vi "DecodificaDO_new.vi"(0 "Array":T7[](array[typedef]), 7 "DO PLCs in":T5, 9 "statoDO Cdaq in":T9, 11 "DO interfaccia in":T6) -> (6 "Exit?":bool, 8 "DO PLCs out":T4, 10 "statoDO Cdaq out":T9, 15 "DO interfaccia out":T6)   [LabVIEW 2019]
uses:
  controls/statoDO_Cdaq.ctl
  cDAQ/SET SINGLE DO.ctl
  cDAQ/DO List.ctl
  TypeDef/DOinterfaccia.ctl
  ST1200_LIST_IO/StatoDO_PLC_1.ctl
  ST1200_LIST_IO/StatoDO_PLC_2.ctl
  ST1200_LIST_IO/StatoDO_PLC_3.ctl
  GlobalForzaUscite.vi
  Global_DO_Interfaccia.vi
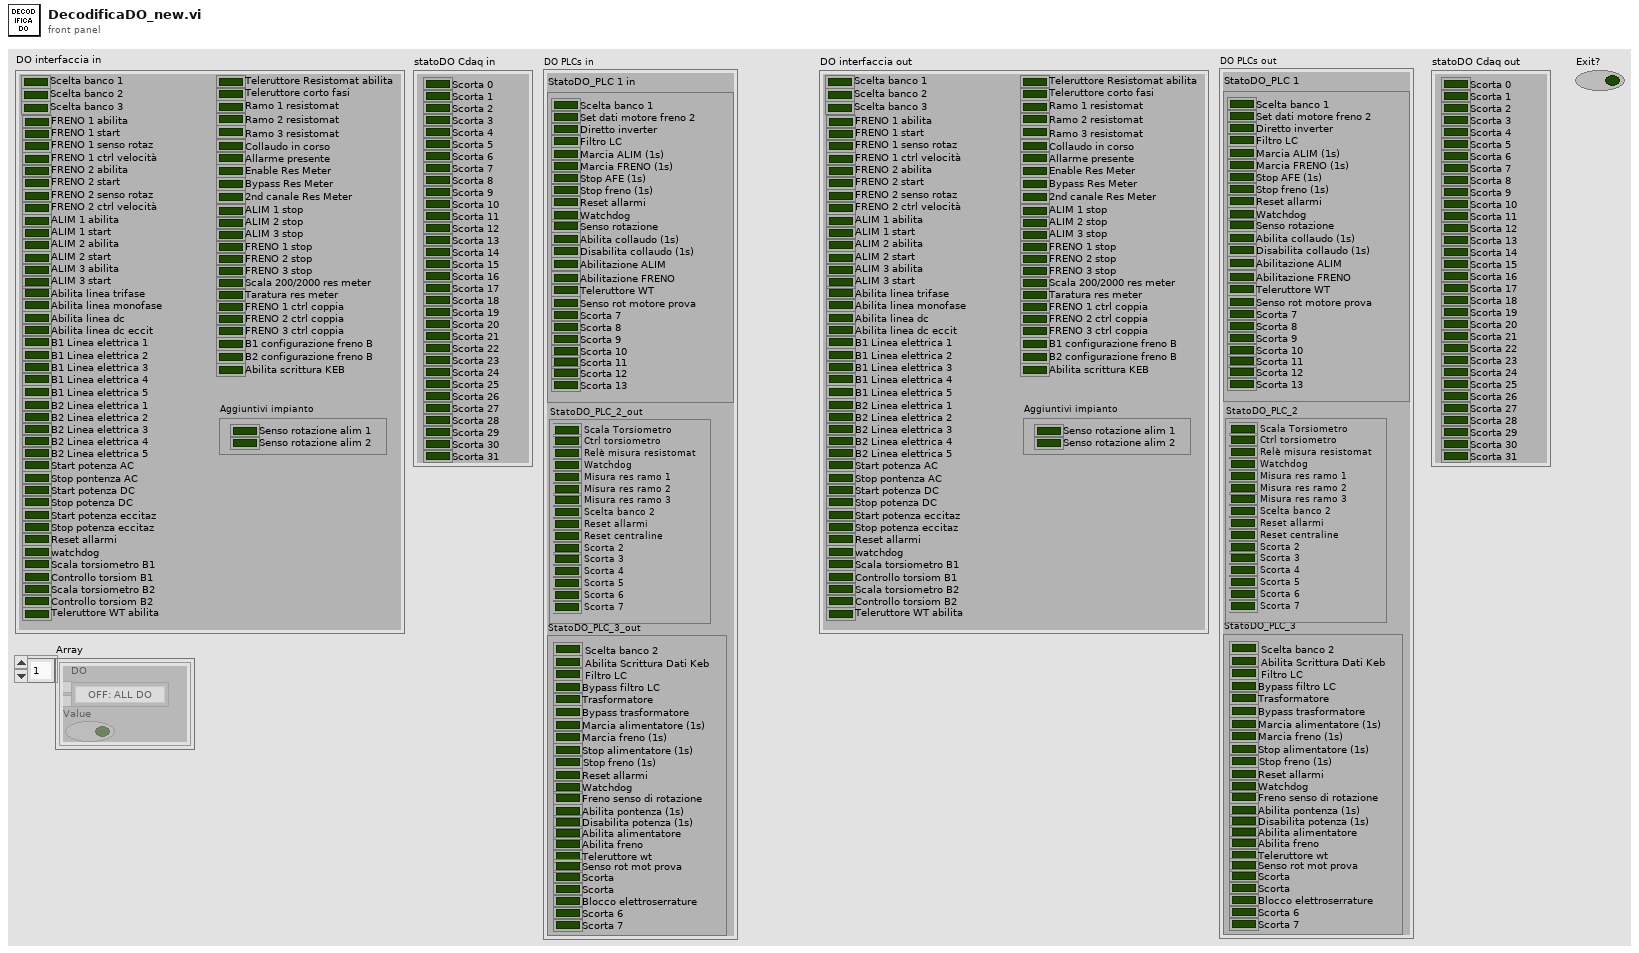
[diagram p1: front panel]
types:
  T1 = typedef "StatoDO_PLC_1.ctl" = cluster{"Scelta banco 1":bool, "Set dati motore freno 2":bool, "Diretto inverter":bool, "Filtro LC":bool, "Marcia ALIM (1s)":bool, "Marcia FRENO (1s)":bool, "Stop AFE (1s)":bool, "Stop freno (1s)":bool, "Reset allarmi":bool, "Watchdog":bool, "Senso rotazione":bool, "Abilita collaudo (1s)":bool, "Disabilita collaudo (1s)":bool, "Abilitazione ALIM":bool, "Abilitazione FRENO":bool, "Teleruttore WT":bool, "Senso rot motore prova":bool, "Scorta 7":bool, "Scorta 8":bool, "Scorta 9":bool, "Scorta 10":bool, "Scorta 11":bool, "Scorta 12":bool, "Scorta 13":bool}
  T2 = typedef "StatoDO_PLC_2.ctl" = cluster{"Scala Torsiometro":bool, "Ctrl torsiometro":bool, "Relè misura resistomat":bool, "Watchdog":bool, "Misura res ramo 1":bool, "Misura res ramo 2":bool, "Misura res ramo 3":bool, "Scelta banco 2":bool, "Reset allarmi":bool, "Reset centraline":bool, "Scorta 2":bool, "Scorta 3":bool, "Scorta 4":bool, "Scorta 5":bool, "Scorta 6":bool, "Scorta 7":bool}
  T3 = typedef "StatoDO_PLC_3.ctl" = cluster{"Scelta banco 2":bool, "Abilita Scrittura Dati Keb":bool, "Filtro LC":bool, "Bypass filtro LC":bool, "Trasformatore":bool, "Bypass trasformatore":bool, "Marcia alimentatore (1s)":bool, "Marcia freno (1s)":bool, "Stop alimentatore (1s)":bool, "Stop freno (1s)":bool, "Reset allarmi":bool, "Watchdog":bool, "Freno senso di rotazione":bool, "Abilita pontenza (1s)":bool, "Disabilita potenza (1s)":bool, "Abilita alimentatore":bool, "Abilita freno":bool, "Teleruttore wt":bool, "Senso rot mot prova":bool, "Scorta":bool, "Scorta":bool, "Blocco elettroserrature":bool, "Scorta 6":bool, "Scorta 7":bool}
  T4 = cluster{"StatoDO_PLC 1":T1, "StatoDO_PLC_2":T2, "StatoDO_PLC_3":T3}
  T5 = cluster{"StatoDO_PLC 1 in":T1, "StatoDO_PLC_2_out":T2, "StatoDO_PLC_3_out":T3}
  T6 = typedef "DOinterfaccia.ctl" = cluster{"Scelta banco 1":bool, "Scelta banco 2":bool, "Scelta banco 3":bool, "FRENO 1 abilita":bool, "FRENO 1 start":bool, "FRENO 1 senso rotaz":bool, "FRENO 1 ctrl velocità":bool, "FRENO 2 abilita":bool, "FRENO 2 start":bool, "FRENO 2 senso rotaz":bool, "FRENO 2 ctrl velocità":bool, "ALIM 1 abilita":bool, "ALIM 1 start":bool, "ALIM 2 abilita":bool, "ALIM 2 start":bool, "ALIM 3 abilita":bool, "ALIM 3 start":bool, "Abilita linea trifase":bool, "Abilita linea monofase":bool, "Abilita linea dc":bool, "Abilita linea dc eccit":bool, "B1 Linea elettrica 1":bool, "B1 Linea elettrica 2":bool, "B1 Linea elettrica 3":bool, "B1 Linea elettrica 4":bool, "B1 Linea elettrica 5":bool, "B2 Linea elettrica 1":bool, "B2 Linea elettrica 2":bool, "B2 Linea elettrica 3":bool, "B2 Linea elettrica 4":bool, "B2 Linea elettrica 5":bool, "Start potenza AC":bool, "Stop pontenza AC":bool, "Start potenza DC":bool, "Stop potenza DC":bool, "Start potenza eccitaz":bool, "Stop potenza eccitaz":bool, "Reset allarmi":bool, "watchdog":bool, "Scala torsiometro B1":bool, "Controllo torsiom B1":bool, "Scala torsiometro B2":bool, "Controllo torsiom B2":bool, "Teleruttore WT abilita":bool, "Teleruttore Resistomat abilita":bool, "Teleruttore corto fasi":bool, "Ramo 1 resistomat":bool, "Ramo 2 resistomat":bool, "Ramo 3 resistomat":bool, "Collaudo in corso":bool, "Allarme presente":bool, "Enable Res Meter":bool, "Bypass Res Meter":bool, "2nd canale Res Meter":bool, "Scala 200/2000 res meter":bool, "Taratura res meter":bool, "FRENO 1 ctrl coppia":bool, "FRENO 2 ctrl coppia":bool, "FRENO 3 ctrl coppia":bool, "Aggiuntivi impianto":cluster{"Senso rotazione alim 1":bool, "Senso rotazione alim 2":bool}, "ALIM 1 stop":bool, "ALIM 2 stop":bool, "ALIM 3 stop":bool, "FRENO 1 stop":bool, "FRENO 2 stop":bool, "FRENO 3 stop":bool, "B1 configurazione freno B":bool, "B2 configurazione freno B":bool, "Abilita scrittura KEB":bool}
  T7 = typedef "SET SINGLE DO.ctl" = cluster{"DO":T8, "Value":bool}
  T8 = typedef "DO List.ctl" = enum16{"OFF: ALL DO", "*ABILITA freno 1", "*ABILITA freno 2", "*ABILITA freno 3", "*START freno 1", "*START freno 2", "*START freno 3", "*STOP freno 1", "*STOP freno 3", "*STOP freno 2", "*Senso rot freno 1", "*Senso rot freno 2", "*Senso rot freno 3", "*Ctrl velocità freno 1", "*Ctrl velocità freno 2", "*Ctrl velocità freno 3", "*Ctrl coppia freno 1", "*Ctrl coppia freno 2", "*Ctrl coppia freno 3", "*ABILITA alimentatore 1", "*ABILITA alimentatore 2", "*ABILITA alimentatore 3", "*ABILITA alimentatore 4", "*START alimentatore 1", "*START alimentatore 2", "*START alimentatore 3", "*START alimentatore 4", "*STOP alimentatore 1", "*STOP alimentatore 2", "*STOP alimentatore 3", "*STOP alimentatore 4", "SENSO ROT alimentatore 1", "SENSO ROT alimentatore 2", "Abilita LEM 1000A", "Abilita LEM 300A", "Abilita sensori EXT WT", "B1 Seleziona linea 1", "B1 Seleziona linea 2", "B1 Seleziona linea 3", "B1 Seleziona linea 4", "B1 Seleziona linea 5", "B2 Seleziona linea 1", "B2 Seleziona linea 2", "B2 Seleziona linea 3", "B2 Seleziona linea 4", "B2 Seleziona linea 5", "*Reset allarmi", "*Start potenza AC", "*Stop potenza AC", "*Start potenza DC", "*Stop potenza DC", "*Start potenza DC eccit", "*Stop pontenza DC eccit", "Bypass res meter", "2nd canale res meter", "Enable res meter", "*Abilit teler ramo WT", "*Abil teler ramo princ Resit", "*Abil teler ramo 1 Resist", "*Abil teler ramo 2 Resist", "*Abil teler ramo 3 Resist", "*Abil cortocirc avvolgim", "*Controllo torsiometro B1", "*Controllo Torsiom B2", "*Scala torsiometro B1", "*Scala torsiometro B2", "*Collaudo in corso", "*Allarme presente", "Abilitazione elettroserratura", "Exit", "*Abilita collaudo", "*Abilita potenza trifase", "*Abilita potenza monofase", "*Abilita potenza DC", "*Abilita potenza DC eccit", "*Disabilita teleruttori potenza", "Set teleruttori prova a freddo", "Prova a freddo monofase", "Watchdog", "Forza DO PLC 3", "Forza DO PLC 2", "Forza DO PLC 1", "Forza DO cDAQ", "Scala 2000(T) 200(F) res meter", "Seleziona banco 1", "Seleziona banco 2", "Comando azionam in blocco", "Comando azionam reset", "Sensibilità freno 16 32 nm", "Reset Allarmi", "Carico res - Ramo 1", "Carico res - Ramo 2", "Carico res - Ramo 3", "Carico res - Ramo 4", "Carico res - Ramo 5", "Carico res - Ramo 6", "Carico res - Ramo 7", "Carico res - Ramo 8", "Carico res - Ramo 9", "Carico res - Ramo 10", "Carico res - Ramo 11", "Carico res - Start ventilatore", "Carico res - Stop ventilatore", "Abilita potenza solo freno", "Abilita AFE + freno trasc", "Abilita potenza carico resistivo", "Chiudi potenza AFE", "Apri potenza AFE", "Start AFE", "Config Banco2 TDE", "Misura diretto WT", "Ripristina centralina protezioni", "Abilita Scrittura Dati Keb"}
  T9 = typedef "statoDO_Cdaq.ctl" = cluster{"Scorta 0":bool, "Scorta 1":bool, "Scorta 2":bool, "Scorta 3":bool, "Scorta 4":bool, "Scorta 5":bool, "Scorta 6":bool, "Scorta 7":bool, "Scorta 8":bool, "Scorta 9":bool, "Scorta 10":bool, "Scorta 11":bool, "Scorta 12":bool, "Scorta 13":bool, "Scorta 14":bool, "Scorta 15":bool, "Scorta 16":bool, "Scorta 17":bool, "Scorta 18":bool, "Scorta 19":bool, "Scorta 20":bool, "Scorta 21":bool, "Scorta 22":bool, "Scorta 23":bool, "Scorta 24":bool, "Scorta 25":bool, "Scorta 26":bool, "Scorta 27":bool, "Scorta 28":bool, "Scorta 29":bool, "Scorta 30":bool, "Scorta 31":bool}
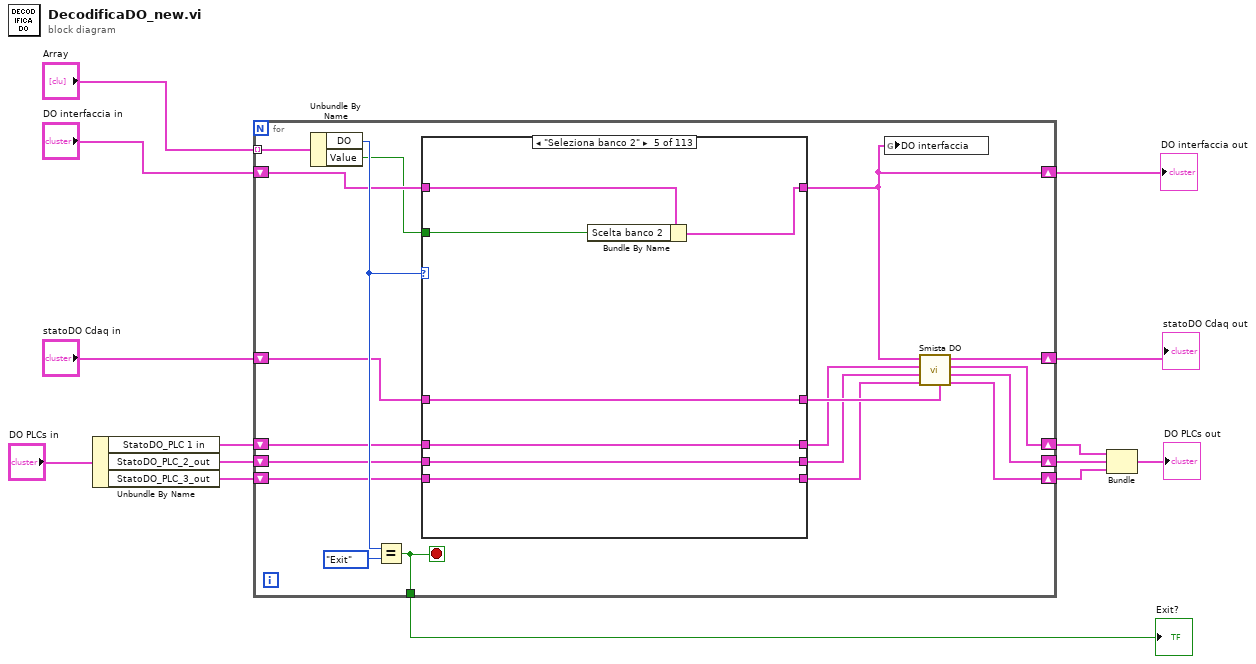
[diagram p0: block diagram]
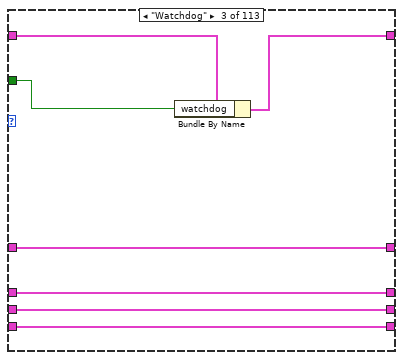
[diagram p4: hidden frame]
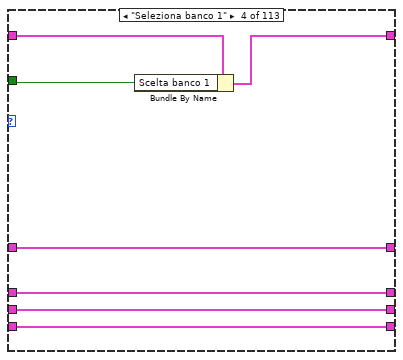
[diagram p5: hidden frame]
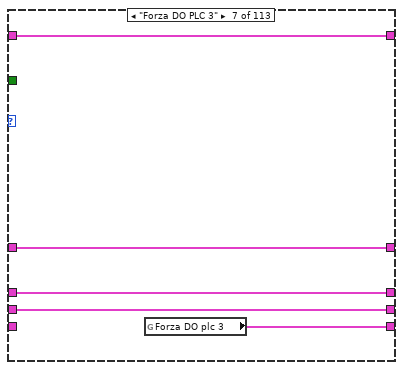
[diagram p7: hidden frame]
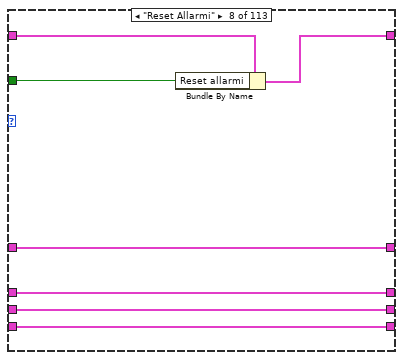
[diagram p8: hidden frame]
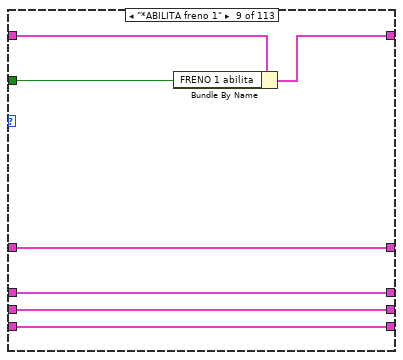
[diagram p9: hidden frame]
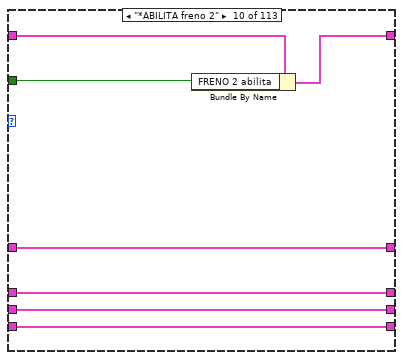
[diagram p10: hidden frame]
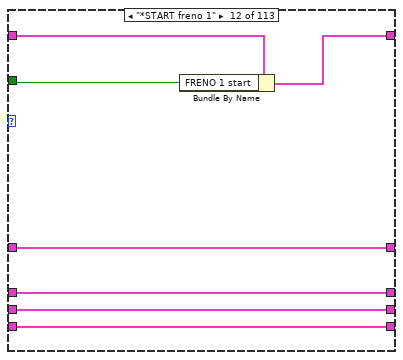
[diagram p12: hidden frame]
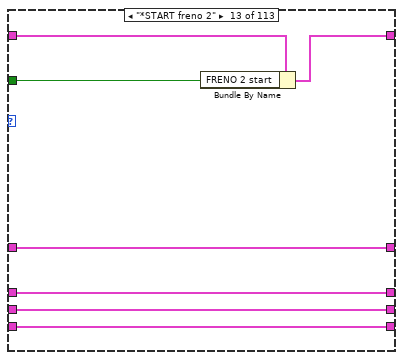
[diagram p13: hidden frame]
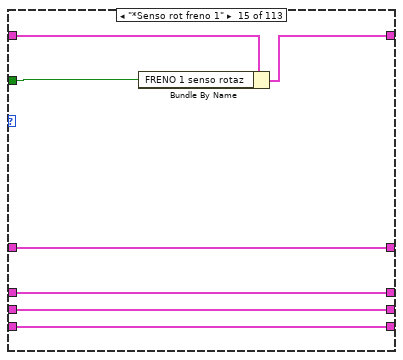
[diagram p15: hidden frame]
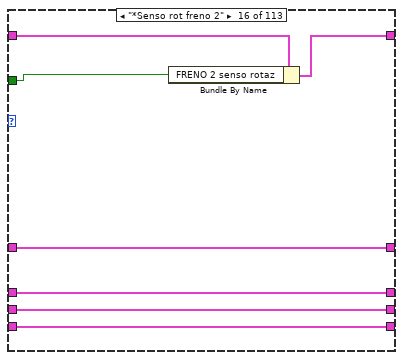
[diagram p16: hidden frame]
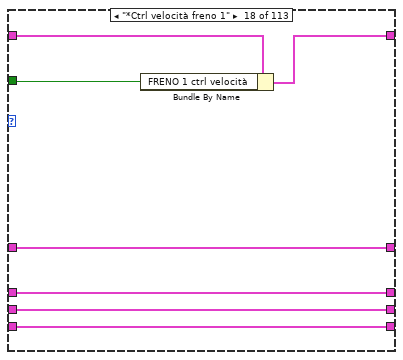
[diagram p18: hidden frame]
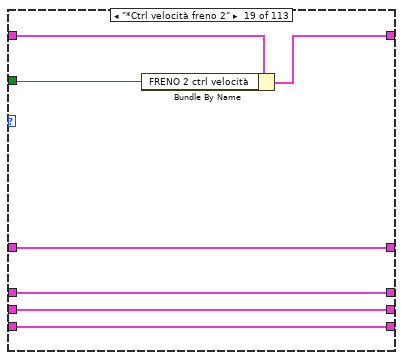
[diagram p19: hidden frame]
diagram:
  n1 = Unbundle By Name("DO PLCs in") -> ("StatoDO_PLC 1 in"=w7:T1, "StatoDO_PLC_2_out"=w6:T2, "StatoDO_PLC_3_out"=w5:T3)
  n2 = for {
    tunnel: "Array" -> [w33] mode=indexing
    shift-right: [w30] -> w11
    shift-left: "statoDO Cdaq in" -> [w24]
    tunnel: [w32] -> w14
    shift-right: [w22] -> w4
    shift-left: w7 -> [w25]
    shift-right: [w23] -> w9
    shift-left: "DO interfaccia in" -> [w27]
    shift-right: [w20] -> w3
    shift-left: w6 -> [w17]
    shift-right: [w19] -> w2
    shift-left: w5 -> [w18]
    stop <- w32 stop-if-true
    n3 = Unbundle By Name(w33) -> ("DO"=w29:T8, "Value"=w26:bool)
    n4 = Equal?(x=w29, y=DO_List."Exit" ("DO")) -> (x = y?=w32:bool)
    n5 = case shown="\"Seleziona banco 2\"" w29 {
      tunnel: [w37 w42 w49 w56 w63 w68 w71 w80 w87 w94 w99 w106 w113 w118 w125 w132 w137 w144 w151 w156 w163 w170 w177 w182 w189 w196 w203 w208 w216 w224 w232 w240 w248 w255 w262 w269 w276 w283 w288 w293 w300 w307 w314 w321 w328 w335 w342 w349 w356 w363 w370 w377 w384 w389 w394 w402 w410 w418 w426 w433 w441 w446 w453 w460 w467 w474 w481 w488 w493 w498 w503 w508 w509 w518 w523 w528 w533 w538 w543 w548 w553 w558 w563 w568 w575 w580 w585 w590 w595 w600 w605 w610 w615 w622 w627 w632 w639 w646 w653 w660 w667 w674 w681 w688 w693 w700 w707 w715 w723 w731 w739 w747 w754] -> w28
      tunnel: [w36 w41 w48 w55 w62 w67 w69 w79 w86 w93 w98 w105 w112 w117 w124 w131 w136 w143 w150 w155 w162 w169 w176 w181 w188 w195 w202 w207 w215 w223 w231 w239 w247 w254 w261 w268 w275 w282 w287 w292 w299 w306 w313 w320 w327 w334 w341 w348 w355 w362 w369 w376 w383 w388 w393 w401 w409 w417 w425 w432 w440 w445 w452 w459 w466 w473 w480 w487 w492 w497 w502 w504 w513 w517 w522 w527 w532 w537 w542 w547 w552 w557 w562 w567 w574 w579 w584 w589 w594 w599 w604 w609 w614 w621 w626 w631 w638 w645 w652 w659 w666 w673 w680 w687 w692 w699 w706 w714 w722 w730 w738 w746 w753] -> w21
      tunnel: [_ w40 w46 w53 w58 w64 w73 w77 w83 w91 w97 w102 w110 w116 w122 w129 w135 w141 w148 w154 w160 w167 w174 w180 w186 w193 w200 w206 w213 w220 w229 w237 w245 w252 w259 w264 w273 w278 w284 w289 w297 w304 w311 w318 w325 w332 w339 w345 w353 w360 w366 w374 w381 w385 w392 w399 w405 w413 w421 w430 w438 w444 w450 w457 w464 w470 w478 w485 w489 w494 w501 w507 w512 w514 w519 w524 w529 w534 w539 w544 w549 w554 w559 w564 w570 w576 w581 w586 w591 w596 w601 w606 w611 w616 w623 w628 w634 w641 w647 w655 w662 w668 w675 w682 w691 w695 w702 w710 w718 w726 w734 w742 w748] -> w23
      tunnel: w27 -> [_ w40 w47 w54 w59 w64 w73 w78 w85 w92 w97 w103 w111 w116 w123 w130 w135 w142 w149 w154 w161 w168 w175 w180 w187 w194 w201 w206 w214 w221 w230 w238 w246 w253 w260 w265 w274 w279 w284 w289 w298 w305 w312 w319 w326 w333 w340 w346 w354 w361 w367 w375 w382 w385 w392 w400 w406 w414 w422 w431 w439 w444 w451 w458 w465 w471 w479 w486 w489 w494 w501 w507 w512 w514 w519 w524 w529 w534 w539 w544 w549 w554 w559 w564 w571 w576 w581 w586 w591 w596 w601 w606 w611 w617 w623 w628 w635 w642 w649 w656 w663 w670 w676 w683 w691 w696 w703 w711 w719 w727 w735 w743 w750]
      tunnel: w26 -> [_ _ w45 w52 w57 _ _ w74 w84 w90 _ w104 w109 _ w121 w128 _ w140 w147 _ w159 w166 w173 _ w185 w192 w199 _ w212 w222 w228 w236 w244 w249 w258 w263 w272 w277 _ _ w296 w303 w310 w317 w324 w331 w338 w347 w352 w359 w368 w373 w380 _ _ w398 w404 w412 w420 _ _ _ w449 w456 w463 w472 w477 w484 _ _ _ _ _ _ _ _ _ _ _ _ _ _ _ _ _ _ _ _ _ _ _ _ _ w618 _ _ w633 w640 w648 w654 w661 w669 w677 w684 _ w694 w701 w709 w716 w724 w732 w740 w749]
      tunnel: w25 -> [w36 w41 w48 w55 w62 w67 w69 w79 w86 w93 w98 w105 w112 w117 w124 w131 w136 w143 w150 w155 w162 w169 w176 w181 w188 w195 w202 w207 w215 w223 w231 w239 w247 w254 w261 w268 w275 w282 w287 w292 w299 w306 w313 w320 w327 w334 w341 w348 w355 w362 w369 w376 w383 w388 w393 w401 w409 w417 w425 w432 w440 w445 w452 w459 w466 w473 w480 w487 w492 w497 w502 _ w513 w517 w522 w527 w532 w537 w542 w547 w552 w557 w562 w567 w574 w579 w584 w589 w594 w599 w604 w609 w614 w621 w626 w631 w638 w645 w652 w659 w666 w673 w680 w687 w692 w699 w706 w714 w722 w730 w738 w746 w753]
      tunnel: w24 -> [w37 w42 w49 w56 w63 w68 w71 w80 w87 w94 w99 w106 w113 w118 w125 w132 w137 w144 w151 w156 w163 w170 w177 w182 w189 w196 w203 w208 w216 w224 w232 w240 w248 w255 w262 w269 w276 w283 w288 w293 w300 w307 w314 w321 w328 w335 w342 w349 w356 w363 w370 w377 w384 w389 w394 w402 w410 w418 w426 w433 w441 w446 w453 w460 w467 w474 w481 w488 w493 w498 w503 w508 _ w518 w523 w528 w533 w538 w543 w548 w553 w558 w563 w568 w575 w580 w585 w590 w595 w600 w605 w610 w615 w622 w627 w632 w639 w646 w653 w660 w667 w674 w681 w688 w693 w700 w707 w715 w723 w731 w739 w747 w754]
      tunnel: w18 -> [w34 w38 w43 w50 w60 w65 _ w75 w81 w88 w95 w100 w107 w114 w119 w126 w133 w138 w145 w152 w157 w164 w171 w178 w183 w190 w197 w204 w209 w217 w225 w233 w241 w250 w256 w266 w270 w280 w285 w290 w294 w301 w308 w315 w322 w329 w336 w343 w350 w357 w364 w371 w378 w386 w390 w396 w407 w415 w423 w428 w434 w442 w447 w454 w461 w468 w475 w482 w490 w495 w500 w505 w510 w515 w520 w525 w530 w535 w540 w545 w550 w555 w560 w565 w572 w577 w582 w587 w592 w597 w602 w607 w612 w619 w624 w629 w636 w643 w650 w657 w664 w671 w678 w685 w689 w697 w704 w712 w720 w728 w736 w744 w751]
      tunnel: w17 -> [w35 w39 w44 w51 w61 w66 w72 w76 w82 w89 w96 w101 w108 w115 w120 w127 w134 w139 w146 w153 w158 w165 w172 w179 w184 w191 w198 w205 w210 w218 w226 w234 w242 w251 w257 w267 w271 w281 w286 w291 w295 w302 w309 w316 w323 w330 w337 w344 w351 w358 w365 w372 w379 w387 w391 w397 w408 w416 w424 w429 w435 w443 w448 w455 w462 w469 w476 w483 w491 w496 _ w506 w511 w516 w521 w526 w531 w536 w541 w546 w551 w556 w561 w566 w573 w578 w583 w588 w593 w598 w603 w608 w613 w620 w625 w630 w637 w644 w651 w658 w665 w672 w679 w686 w690 w698 w705 w713 w721 w729 w737 w745 w752]
      tunnel: [w35 w39 w44 w51 w61 w66 w72 w76 w82 w89 w96 w101 w108 w115 w120 w127 w134 w139 w146 w153 w158 w165 w172 w179 w184 w191 w198 w205 w210 w218 w226 w234 w242 w251 w257 w267 w271 w281 w286 w291 w295 w302 w309 w316 w323 w330 w337 w344 w351 w358 w365 w372 w379 w387 w391 w397 w408 w416 w424 w429 w435 w443 w448 w455 w462 w469 w476 w483 w491 w496 w499 w506 w511 w516 w521 w526 w531 w536 w541 w546 w551 w556 w561 w566 w573 w578 w583 w588 w593 w598 w603 w608 w613 w620 w625 w630 w637 w644 w651 w658 w665 w672 w679 w686 w690 w698 w705 w713 w721 w729 w737 w745 w752] -> w16
      tunnel: [w34 w38 w43 w50 w60 w65 w70 w75 w81 w88 w95 w100 w107 w114 w119 w126 w133 w138 w145 w152 w157 w164 w171 w178 w183 w190 w197 w204 w209 w217 w225 w233 w241 w250 w256 w266 w270 w280 w285 w290 w294 w301 w308 w315 w322 w329 w336 w343 w350 w357 w364 w371 w378 w386 w390 w396 w407 w415 w423 w428 w434 w442 w447 w454 w461 w468 w475 w482 w490 w495 w500 w505 w510 w515 w520 w525 w530 w535 w540 w545 w550 w555 w560 w565 w572 w577 w582 w587 w592 w597 w602 w607 w612 w619 w624 w629 w636 w643 w650 w657 w664 w671 w678 w685 w689 w697 w704 w712 w720 w728 w736 w744 w751] -> w15
      frame "OFF: ALL DO", Default {
      }
      frame "Exit" {
      }
      frame "Watchdog" {
        n6 = Bundle By Name(cluster=w47, "watchdog"=w45) -> (w46:T6)
      }
      frame "Seleziona banco 1" {
        n7 = Bundle By Name(cluster=w54, "Scelta banco 1"=w52) -> (w53:T6)
      }
      frame "Seleziona banco 2" {
        n8 = Bundle By Name(cluster=w59, "Scelta banco 2"=w57) -> (w58:T6)
      }
      frame "Comando azionam in blocco" {
      }
      frame "Forza DO PLC 3" {
        n9 = global read "GlobalForzaUscite.vi" "Forza DO plc 3"() -> (w70:T3)
      }
      frame "Reset Allarmi" {
        n10 = Bundle By Name(cluster=w78, "Reset allarmi"=w74) -> (w77:T6)
      }
      frame "*ABILITA freno 1" {
        n11 = Bundle By Name(cluster=w85, "FRENO 1 abilita"=w84) -> (w83:T6)
      }
      frame "*ABILITA freno 2" {
        n12 = Bundle By Name(cluster=w92, "FRENO 2 abilita"=w90) -> (w91:T6)
      }
      frame "*ABILITA freno 3" {
      }
      frame "*START freno 1" {
        n13 = Bundle By Name(cluster=w103, "FRENO 1 start"=w104) -> (w102:T6)
      }
      frame "*START freno 2" {
        n14 = Bundle By Name(cluster=w111, "FRENO 2 start"=w109) -> (w110:T6)
      }
      frame "*START freno 3" {
      }
      frame "*Senso rot freno 1" {
        n15 = Bundle By Name(cluster=w123, "FRENO 1 senso rotaz"=w121) -> (w122:T6)
      }
      frame "*Senso rot freno 2" {
        n16 = Bundle By Name(cluster=w130, "FRENO 2 senso rotaz"=w128) -> (w129:T6)
      }
      frame "*Senso rot freno 3" {
      }
      frame "*Ctrl velocità freno 1" {
        n17 = Bundle By Name(cluster=w142, "FRENO 1 ctrl velocità"=w140) -> (w141:T6)
      }
      frame "*Ctrl velocità freno 2" {
        n18 = Bundle By Name(cluster=w149, "FRENO 2 ctrl velocità"=w147) -> (w148:T6)
      }
      frame "*Ctrl velocità freno 3" {
      }
      frame "*ABILITA alimentatore 1" {
        n19 = Bundle By Name(cluster=w161, "ALIM 1 abilita"=w159) -> (w160:T6)
      }
      frame "*ABILITA alimentatore 2" {
        n20 = Bundle By Name(cluster=w168, "ALIM 2 abilita"=w166) -> (w167:T6)
      }
      frame "*ABILITA alimentatore 3" {
        n21 = Bundle By Name(cluster=w175, "ALIM 3 abilita"=w173) -> (w174:T6)
      }
      frame "*ABILITA alimentatore 4" {
      }
      frame "*START alimentatore 1" {
        n22 = Bundle By Name(cluster=w187, "ALIM 1 start"=w185) -> (w186:T6)
      }
      frame "*START alimentatore 2" {
        n23 = Bundle By Name(cluster=w194, "ALIM 2 start"=w192) -> (w193:T6)
      }
      frame "*START alimentatore 3" {
        n24 = Bundle By Name(cluster=w201, "ALIM 3 start"=w199) -> (w200:T6)
      }
      frame "*START alimentatore 4" {
      }
      frame "B1 Seleziona linea 1" {
        w211 = FALSE ("Linea elettrica 5")
        n25 = Bundle By Name(cluster=w214, "B1 Linea elettrica 1"=w212, "B1 Linea elettrica 2"=w211, "B1 Linea elettrica 3"=w211, "B1 Linea elettrica 4"=w211, "B1 Linea elettrica 5"=w211) -> (w213:T6)
      }
      frame "B1 Seleziona linea 2" {
        w219 = FALSE ("Linea elettrica 1")
        n26 = Bundle By Name(cluster=w221, "B1 Linea elettrica 1"=w219, "B1 Linea elettrica 2"=w222, "B1 Linea elettrica 3"=w219, "B1 Linea elettrica 4"=w219, "B1 Linea elettrica 5"=w219) -> (w220:T6)
      }
      frame "B1 Seleziona linea 3" {
        w227 = FALSE ("Linea elettrica 1")
        n27 = Bundle By Name(cluster=w230, "B1 Linea elettrica 1"=w227, "B1 Linea elettrica 2"=w227, "B1 Linea elettrica 3"=w228, "B1 Linea elettrica 4"=w227, "B1 Linea elettrica 5"=w227) -> (w229:T6)
      }
      frame "B1 Seleziona linea 4" {
        w235 = FALSE ("Linea elettrica 5")
        n28 = Bundle By Name(cluster=w238, "B1 Linea elettrica 1"=w235, "B1 Linea elettrica 2"=w235, "B1 Linea elettrica 3"=w235, "B1 Linea elettrica 4"=w236, "B1 Linea elettrica 5"=w235) -> (w237:T6)
      }
      frame "B1 Seleziona linea 5" {
        w243 = FALSE ("Linea elettrica 1")
        n29 = Bundle By Name(cluster=w246, "B1 Linea elettrica 1"=w243, "B1 Linea elettrica 2"=w243, "B1 Linea elettrica 3"=w243, "B1 Linea elettrica 4"=w243, "B1 Linea elettrica 5"=w244) -> (w245:T6)
      }
      frame "*Reset allarmi" {
        n30 = Bundle By Name(cluster=w253, "Reset allarmi"=w249) -> (w252:T6)
      }
      frame "*Start potenza AC" {
        n31 = Bundle By Name(cluster=w260, "Start potenza AC"=w258) -> (w259:T6)
      }
      frame "*Stop potenza AC" {
        n32 = Bundle By Name(cluster=w265, "Stop pontenza AC"=w263) -> (w264:T6)
      }
      frame "*Start potenza DC" {
        n33 = Bundle By Name(cluster=w274, "Start potenza DC"=w272) -> (w273:T6)
      }
      frame "*Stop potenza DC" {
        n34 = Bundle By Name(cluster=w279, "Stop potenza DC"=w277) -> (w278:T6)
      }
      frame "*Start potenza DC eccit" {
      }
      frame "*Stop pontenza DC eccit" {
      }
      frame "Bypass res meter" {
        n35 = Bundle By Name(cluster=w298, "Bypass Res Meter"=w296) -> (w297:T6)
      }
      frame "*Abilit teler ramo WT" {
        n36 = Bundle By Name(cluster=w305, "Teleruttore WT abilita"=w303) -> (w304:T6)
      }
      frame "*Abil teler ramo princ Resit" {
        n37 = Bundle By Name(cluster=w312, "Teleruttore Resistomat abilita"=w310) -> (w311:T6)
      }
      frame "*Abil teler ramo 1 Resist" {
        n38 = Bundle By Name(cluster=w319, "Ramo 1 resistomat"=w317) -> (w318:T6)
      }
      frame "*Abil teler ramo 2 Resist" {
        n39 = Bundle By Name(cluster=w326, "Ramo 2 resistomat"=w324) -> (w325:T6)
      }
      frame "*Abil teler ramo 3 Resist" {
        n40 = Bundle By Name(cluster=w333, "Ramo 3 resistomat"=w331) -> (w332:T6)
      }
      frame "*Abil cortocirc avvolgim" {
        n41 = Bundle By Name(cluster=w340, "Teleruttore corto fasi"=w338) -> (w339:T6)
      }
      frame "*Controllo torsiometro B1" {
        n42 = Bundle By Name(cluster=w346, "Controllo torsiom B1"=w347) -> (w345:T6)
      }
      frame "*Controllo Torsiom B2" {
        n43 = Bundle By Name(cluster=w354, "Controllo torsiom B2"=w352) -> (w353:T6)
      }
      frame "*Scala torsiometro B1" {
        n44 = Bundle By Name(cluster=w361, "Scala torsiometro B1"=w359) -> (w360:T6)
      }
      frame "*Scala torsiometro B2" {
        n45 = Bundle By Name(cluster=w367, "Scala torsiometro B2"=w368) -> (w366:T6)
      }
      frame "*Collaudo in corso" {
        n46 = Bundle By Name(cluster=w375, "Collaudo in corso"=w373) -> (w374:T6)
      }
      frame "*Allarme presente" {
        n47 = Bundle By Name(cluster=w382, "Allarme presente"=w380) -> (w381:T6)
      }
      frame "Abilitazione elettroserratura" {
      }
      frame "*Abilita collaudo" {
      }
      frame "*Abilita potenza trifase" {
        w395 = FALSE ("Abilita linea monofase")
        n48 = Bundle By Name(cluster=w400, "Abilita linea trifase"=w398, "Abilita linea monofase"=w395, "Abilita linea dc"=w395, "Abilita linea dc eccit"=w395) -> (w399:T6)
      }
      frame "*Abilita potenza monofase" {
        w403 = FALSE ("Abilita linea trifase")
        n49 = Bundle By Name(cluster=w406, "Abilita linea trifase"=w403, "Abilita linea monofase"=w404, "Abilita linea dc"=w403, "Abilita linea dc eccit"=w403) -> (w405:T6)
      }
      frame "*Abilita potenza DC" {
        w411 = FALSE ("Abilita linea trifase")
        n50 = Bundle By Name(cluster=w414, "Abilita linea trifase"=w411, "Abilita linea monofase"=w411, "Abilita linea dc"=w412, "Abilita linea dc eccit"=w411) -> (w413:T6)
      }
      frame "*Abilita potenza DC eccit" {
        w419 = FALSE ("Aggiuntivi impianto.Abilita carico resistivo")
        n51 = Bundle By Name(cluster=w422, "Abilita linea trifase"=w419, "Abilita linea monofase"=w419, "Abilita linea dc"=w419, "Abilita linea dc eccit"=w420) -> (w421:T6)
      }
      frame "*Disabilita teleruttori potenza" {
        w427 = FALSE ("Start potenza AC")
        n52 = Bundle By Name(cluster=w431, "Start potenza AC"=w427, "Stop pontenza AC"=w427, "Start potenza DC"=w427, "Stop potenza DC"=w427, "Start potenza eccitaz"=w427, "Stop potenza eccitaz"=w427, "Abilita linea trifase"=w427, "Abilita linea monofase"=w427, "Abilita linea dc"=w427, "Abilita linea dc eccit"=w427) -> (w430:T6)
      }
      frame "Set teleruttori prova a freddo" {
        n53 = Bundle By Name(cluster=w439, "Teleruttore Resistomat abilita"=TRUE, "Teleruttore WT abilita"=FALSE) -> (w438:T6)
      }
      frame "Prova a freddo monofase" {
      }
      frame "2nd canale res meter" {
        n54 = Bundle By Name(cluster=w451, "2nd canale Res Meter"=w449) -> (w450:T6)
      }
      frame "Enable res meter" {
        n55 = Bundle By Name(cluster=w458, "Enable Res Meter"=w456) -> (w457:T6)
      }
      frame "Scala 2000(T) 200(F) res meter" {
        n56 = Bundle By Name(cluster=w465, "Scala 200/2000 res meter"=w463) -> (w464:T6)
      }
      frame "*Ctrl coppia freno 1" {
        n57 = Bundle By Name(cluster=w471, "FRENO 1 ctrl coppia"=w472) -> (w470:T6)
      }
      frame "*Ctrl coppia freno 2" {
        n58 = Bundle By Name(cluster=w479, "FRENO 2 ctrl coppia"=w477) -> (w478:T6)
      }
      frame "*Ctrl coppia freno 3" {
        n59 = Bundle By Name(cluster=w486, "FRENO 3 ctrl coppia"=w484) -> (w485:T6)
      }
      frame "Comando azionam reset" {
      }
      frame "Sensibilità freno 16 32 nm" {
      }
      frame "Forza DO PLC 2" {
        n60 = global read "GlobalForzaUscite.vi" "Forza DO plc 2"() -> (w499:T2)
      }
      frame "Forza DO PLC 1" {
        n61 = global read "GlobalForzaUscite.vi" "Forza DO plc 1"() -> (w504:T1)
      }
      frame "Forza DO cDAQ" {
        n62 = global read "GlobalForzaUscite.vi" "ForzaDO_Cdaq"() -> (w509:T9)
      }
      frame "Carico res - Ramo 1" {
      }
      frame "Carico res - Ramo 2" {
      }
      frame "Carico res - Ramo 3" {
      }
      frame "Carico res - Ramo 4" {
      }
      frame "Carico res - Ramo 5" {
      }
      frame "Carico res - Ramo 6" {
      }
      frame "Carico res - Ramo 7" {
      }
      frame "Carico res - Ramo 8" {
      }
      frame "Carico res - Ramo 9" {
      }
      frame "Carico res - Ramo 10" {
      }
      frame "Carico res - Ramo 11" {
      }
      frame "Abilita potenza solo freno" {
        w569 = FALSE ("Abilita carico resistivo")
        n63 = Bundle By Name(cluster=w571, "Abilita linea trifase"=w569, "Abilita linea monofase"=w569, "Abilita linea dc"=w569, "Abilita linea dc eccit"=w569) -> (w570:T6)
      }
      frame "Abilita potenza carico resistivo" {
      }
      frame "Abilita AFE + freno trasc" {
      }
      frame "Ripristina centralina protezioni" {
      }
      frame "Carico res - Start ventilatore" {
      }
      frame "Carico res - Stop ventilatore" {
      }
      frame "Chiudi potenza AFE" {
      }
      frame "Start AFE" {
      }
      frame "Apri potenza AFE" {
      }
      frame "Abilita LEM 1000A" {
        n64 = Bundle By Name(cluster=w617, "Aggiuntivi impianto.Senso rotazione alim 2"=w618) -> (w616:T6)
      }
      frame "Abilita LEM 300A" {
      }
      frame "Abilita sensori EXT WT" {
      }
      frame "Config Banco2 TDE" {
        n65 = Bundle By Name(cluster=w635, "B1 configurazione freno B"=w633, "B2 configurazione freno B"=w633) -> (w634:T6)
      }
      frame "Misura diretto WT" {
        n66 = Bundle By Name(cluster=w642, "Aggiuntivi impianto.Senso rotazione alim 1"=w640) -> (w641:T6)
      }
      frame "*STOP freno 1" {
        n67 = Bundle By Name(cluster=w649, "FRENO 1 stop"=w648) -> (w647:T6)
      }
      frame "*STOP freno 3" {
        n68 = Bundle By Name(cluster=w656, "FRENO 3 stop"=w654) -> (w655:T6)
      }
      frame "*STOP freno 2" {
        n69 = Bundle By Name(cluster=w663, "FRENO 2 stop"=w661) -> (w662:T6)
      }
      frame "*STOP alimentatore 1" {
        n70 = Bundle By Name(cluster=w670, "ALIM 1 stop"=w669) -> (w668:T6)
      }
      frame "*STOP alimentatore 2" {
        n71 = Bundle By Name(cluster=w676, "ALIM 2 stop"=w677) -> (w675:T6)
      }
      frame "*STOP alimentatore 3" {
        n72 = Bundle By Name(cluster=w683, "ALIM 3 stop"=w684) -> (w682:T6)
      }
      frame "*STOP alimentatore 4" {
      }
      frame "SENSO ROT alimentatore 1" {
        n73 = Bundle By Name(cluster=w696, "Aggiuntivi impianto.Senso rotazione alim 1"=w694) -> (w695:T6)
      }
      frame "SENSO ROT alimentatore 2" {
        n74 = Bundle By Name(cluster=w703, "Aggiuntivi impianto.Senso rotazione alim 2"=w701) -> (w702:T6)
      }
      frame "B2 Seleziona linea 1" {
        w708 = FALSE ("B1 Linea elettrica 2")
        n75 = Bundle By Name(cluster=w711, "B2 Linea elettrica 1"=w709, "B2 Linea elettrica 2"=w708, "B2 Linea elettrica 3"=w708, "B2 Linea elettrica 4"=w708, "B2 Linea elettrica 5"=w708) -> (w710:T6)
      }
      frame "B2 Seleziona linea 2" {
        w717 = FALSE ("B1 Linea elettrica 2")
        n76 = Bundle By Name(cluster=w719, "B2 Linea elettrica 1"=w717, "B2 Linea elettrica 2"=w716, "B2 Linea elettrica 3"=w717, "B2 Linea elettrica 4"=w717, "B2 Linea elettrica 5"=w717) -> (w718:T6)
      }
      frame "B2 Seleziona linea 3" {
        w725 = FALSE ("B1 Linea elettrica 2")
        n77 = Bundle By Name(cluster=w727, "B2 Linea elettrica 1"=w725, "B2 Linea elettrica 2"=w725, "B2 Linea elettrica 3"=w724, "B2 Linea elettrica 4"=w725, "B2 Linea elettrica 5"=w725) -> (w726:T6)
      }
      frame "B2 Seleziona linea 4" {
        w733 = FALSE ("B1 Linea elettrica 2")
        n78 = Bundle By Name(cluster=w735, "B2 Linea elettrica 1"=w733, "B2 Linea elettrica 2"=w733, "B2 Linea elettrica 3"=w733, "B2 Linea elettrica 4"=w732, "B2 Linea elettrica 5"=w733) -> (w734:T6)
      }
      frame "B2 Seleziona linea 5" {
        w741 = FALSE ("B1 Linea elettrica 2")
        n79 = Bundle By Name(cluster=w743, "B2 Linea elettrica 1"=w741, "B2 Linea elettrica 2"=w741, "B2 Linea elettrica 3"=w741, "B2 Linea elettrica 4"=w741, "B2 Linea elettrica 5"=w740) -> (w742:T6)
      }
      frame "Abilita Scrittura Dati Keb" {
        n80 = Bundle By Name(cluster=w750, "Abilita scrittura KEB"=w749) -> (w748:T6)
      }
    }
    n81 = global write "Global_DO_Interfaccia.vi" "DO interfaccia"(w23) -> ()
    n82 = call "Smista DO.vi"("Forza DO Cdaq"=w28, "Forza DO plc 3"=w15, "Forza DO plc 2"=w16, "Forza DO plc 1"=w21, "DO interfaccia in"=w23) -> ("StatoDO_PLC_3_out"=w19:T3, "StatoDO_PLC_2_out"=w20:T2, "StatoDO_PLC_1_out"=w22:T1, "statoDO Cdaq out"=w30:T9)  [unwired: 3 in]
  }
  "statoDO Cdaq out" <- w11
  "Exit?" <- w14
  "DO interfaccia out" <- w9
  n83 = Bundle("StatoDO_PLC 1 in"=w4, "StatoDO_PLC_2_out"=w3, "StatoDO_PLC_3_out"=w2) -> (→"DO PLCs out":T5)  [unwired: 1 in]
